vi "Kerosene_Weight.vi"() -> ()   [LabVIEW 2018]
panel:
  in  "End Loop":bool
  in  "Temp":dbl
  out "?":dbl
  out "Kerosene Weight":dbl(knob) scale=0.0..150.0
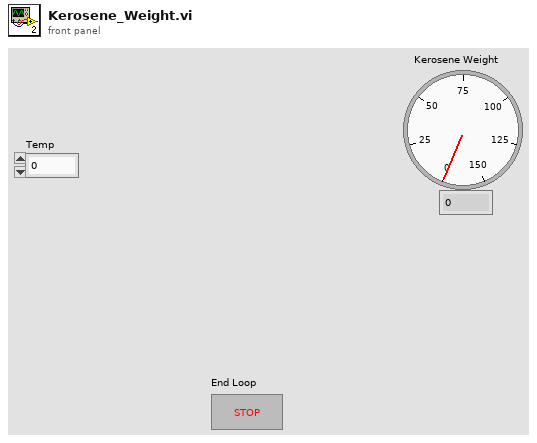
[diagram p1: front panel]
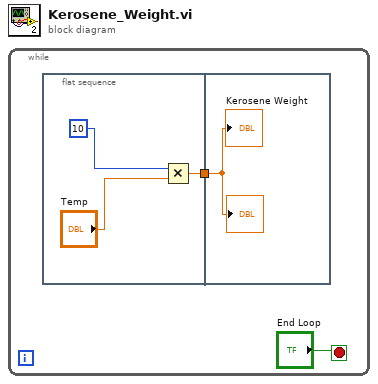
[diagram p0: block diagram]
diagram:
  n1 = while {
    stop <- "End Loop" stop-if-true
    n2 = flat-sequence {
      tunnel: [w3] -> w2
      tunnel: w2 -> [w6]
      frame #0 {
        n3 = Multiply(x=10, y="Temp") -> (x*y=w3:dbl)
      }
      frame #1 {
        "Kerosene Weight" <- w6
        "?" <- w6
      }
    }
  }
